vi "trash_Read Configuration.vi"(8 "error in":errorcluster, 11 "CoreOOB_Rx in":refnum<class "ChanMngOOB_Rx.lvclass">) -> (0 "error out":errorcluster, 2 "Configuration Data":variant, 3 "CoreOOB_Rx out":refnum<class "ChanMngOOB_Rx.lvclass">)   [LabVIEW 2021]
uses:
  ChanMngOOB_Rx.lvclass/ChanMngOOB_Rx.ctl
  ChanMngOOB_Rx.lvclass
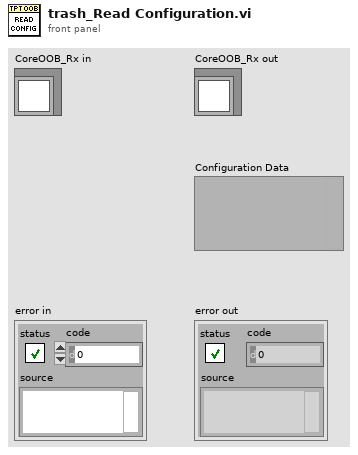
[diagram p1: front panel]
types:
  T1 = typedef "ChanMngOOB_Rx.lvclass/Template Payload.ctl" = cluster{"Connections":T2[], "Forces":T3[]}
  T2 = typedef "ChanMngOOB_Rx.lvclass/Channel Connection Data.ctl" = cluster{"Publisher Name":string, "Subscriber Name":string, "Connection Data":u8[]}
  T3 = typedef "ChanMngOOB_Rx.lvclass/Channel Fault Data.ctl" = cluster{"Channel Name":string, "Force Data":u8[], "Force Active":bool}
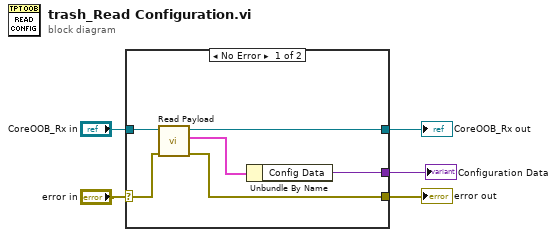
[diagram p0: block diagram]
diagram:
  n1 = case shown="No Error" "error in" {
    selector: "error in" -> [w9 w13]
    tunnel: [w6 w13] -> w5
    tunnel: [w10 w12] -> w4
    tunnel: "CoreOOB_Rx in" -> [w11 w12]
    tunnel: [w7 _] -> w1
    frame No Error {
      n2 = call "Read Payload.vi"("error in"=w9, "CoreOOB_Rx in"=w11) -> ("error out"=w6:errorcluster, "data"=w8:T1, "CoreOOB_Rx out"=w10:refnum<class "ChanMngOOB_Rx.lvclass">)  [unwired: 7 in]
      n3 = Unbundle By Name(w8) -> ("Config Data"=w7:variant)
    }
    frame Error {
    }
  }
  "error out" <- w5
  "CoreOOB_Rx out" <- w4
  "Configuration Data" <- w1
